vi "MGI RWA Replace Characters.vi"(0 "String In":string) -> (2 "String Out":string)   [LabVIEW 2024]
doc: "This VI was created for use with the Read/Write Anything VIs. It converts any carriage returns and line feeds in the string to unique identifier strings which can be converted back upon reading the file.\n\nAuthored by Robert C. Mortensen\nsupport@mooregoodideas.com\nwww.mooregoodideas.com\n\nCopyright (c) 2010, Moore Good Ideas, Inc.\n\nAll rights reserved.\n\nRedistribution and use in source and binary forms, with or without modification, are permitted provided that the following conditions are met:\n\n * Redistributions of source code must retain the above copyright notice, this list of conditions and the following disclaimer.\n * Redistributions in binary form must reproduce the above copyright notice, this list of conditions and the following disclaimer in the documentation and/or other materials provided with the distribution.\n * Neither the name of Moore Good Ideas, Inc. nor the names of its contributors may be used to endorse or promote products derived from this software without specific prior written permission.\n\nTHIS SOFTWARE IS PROVIDED BY THE COPYRIGHT HOLDERS AND CONTRIBUTORS \"AS IS\" AND ANY EXPRESS OR IMPLIED WARRANTIES, INCLUDING, BUT NOT LIMITED TO, THE IMPLIED WARRANTIES OF MERCHANTABILITY AND FITNESS FOR A PARTICULAR PURPOSE ARE DISCLAIMED. IN NO EVENT SHALL THE COPYRIGHT OWNER OR CONTRIBUTORS BE LIABLE FOR ANY DIRECT, INDIRECT, INCIDENTAL, SPECIAL, EXEMPLARY, OR CONSEQUENTIAL DAMAGES (INCLUDING, BUT NOT LIMITED TO, PROCUREMENT OF SUBSTITUTE GOODS OR SERVICES; LOSS OF USE, DATA, OR PROFITS; OR BUSINESS INTERRUPTION) HOWEVER CAUSED AND ON ANY THEORY OF LIABILITY, WHETHER IN CONTRACT, STRICT LIABILITY, OR TORT (INCLUDING NEGLIGENCE OR OTHERWISE) ARISING IN ANY WAY OUT OF THE USE OF THIS SOFTWARE, EVEN IF ADVISED OF THE POSSIBILITY OF SUCH DAMAGE."
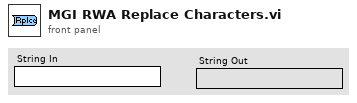
[diagram p1: front panel]
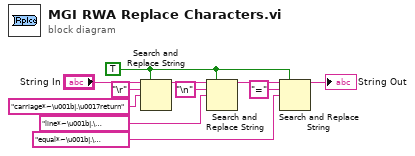
[diagram p0: block diagram]
diagram:
  w3 = TRUE ("replace all? (F)")
  n1 = Search and Replace String(replace all?=w3, input string="String In", search string="\r" ("replace string (\"\")"), replace string="carriage*~\u001b|.\u0017return") -> (result string=w8:string)  [unwired: 4 in, 3 out]
  n2 = Search and Replace String(replace all?=w3, input string=w8, search string="\n" ("replace string (\"\")"), replace string="line*~\u001b|.\u0017feed") -> (result string=w4:string)  [unwired: 4 in, 3 out]
  n3 = Search and Replace String(replace all?=w3, input string=w4, search string="=" ("replace string (\"\")"), replace string="equal*~\u001b|.\u0017sign") -> (result string=→"String Out":string)  [unwired: 4 in, 3 out]
